vi "Modify_Image_Histogram-1.vi"(4 "[IN] Parameter":sgl format="%.2f", 6 "[IN] Operator":T4(ring), 7 "# channel":u8, 8 "error IN":errorcluster, 9 "[IN] Filtering Settings":T2, 11 "[IN] LoG Processed Image":T3) -> (0 "error OUT":errorcluster, 1 "[OUT] Filtering Settings":T2, 2 "[OUT] Histogram":T1 {"Incremental Value" format="%.2f"; "Starting Value" format="%.2f"}, 3 "[OUT] Histogram Modified Image":T3)   [LabVIEW 2013]
doc: "This subVI modifies image through various mathlookup operations (see the built-in function \"IMAQ MathLookup\")"
uses:
  <vilib>/vision/Image Controls.llb/IMAQ Image.ctl
  <vilib>/vision/NI_Vision_Development_Module.lvlib
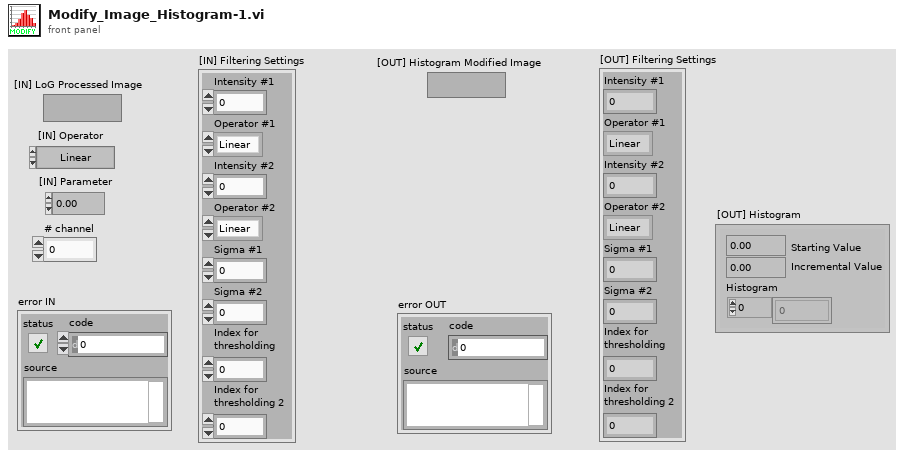
[diagram p1: front panel]
types:
  T1 = cluster{"Starting Value":sgl, "Incremental Value":sgl, "Histogram":u32[]}
  T2 = cluster{"Intensity #1":sgl, "Operator #1":enum32{"Linear", "Log", "Exp", "Square", "Square root", "Power X", "Power 1/X"}, "Intensity #2":sgl, "Operator #2":enum32{"Linear", "Log", "Exp", "Square", "Square root", "Power X", "Power 1/X"}, "Sigma #1":dbl, "Sigma #2":dbl, "Index for \nthresholding":u8, "Index for \nthresholding 2":u8}
  T3 = typedef "IMAQ Image.ctl" = refnum<image>
  T4 = enum32{"Linear", "Log", "Exp", "Square", "Square root", "Power X", "Power 1/X"}
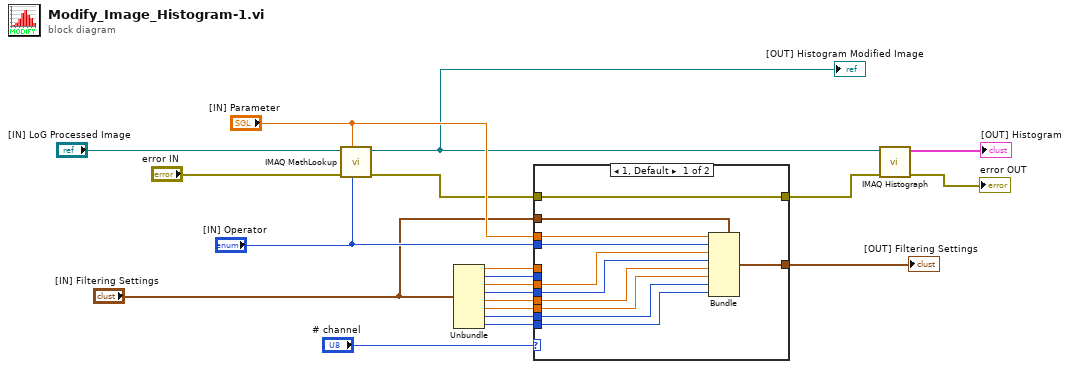
[diagram p0: block diagram]
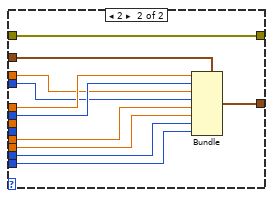
[diagram p2: hidden frame]
diagram:
  n1 = call "IMAQ MathLookup"("Operator"="[IN] Operator", "X Value"="[IN] Parameter", "error in (no error)"="error IN", "Image Src"="[IN] LoG Processed Image") -> ("error out"=w4:errorcluster, "Image Dst Out"=w5:T3)  [unwired: 6 in]
  "[OUT] Histogram Modified Image" <- w5
  n2 = Unbundle("[IN] Filtering Settings") -> ("Intensity #1"=w17:sgl, "Operator #1"=w16:T4, "Intensity #2"=w15:sgl, "Operator #2"=w14:T4, "Sigma #1"=w10:dbl, "Sigma #2"=w9:dbl, "Index for \nthresholding"=w8:u8, "Index for \nthresholding 2"=w7:u8)
  n3 = case shown="1, Default" "# channel" {
    tunnel: w17 -> [_ w41]
    tunnel: w16 -> [_ w40]
    tunnel: w15 -> [w27 _]
    tunnel: w14 -> [w26 _]
    tunnel: "[IN] Parameter" -> [w30 w39]
    tunnel: "[IN] Operator" -> [w28 w38]
    tunnel: "[IN] Filtering Settings" -> [w31 w42]
    tunnel: w10 -> [w25 w35]
    tunnel: w9 -> [w24 w34]
    tunnel: w8 -> [w23 w36]
    tunnel: w7 -> [w22 w37]
    tunnel: [w29 w33] -> w6
    tunnel: w4 -> [w21 w32]
    tunnel: [w21 w32] -> w3
    frame 1, Default {
      n4 = Bundle(cluster=w31, "Intensity #1"=w30, "Operator #1"=w28, "Intensity #2"=w27, "Operator #2"=w26, "Sigma #1"=w25, "Sigma #2"=w24, "Index for \nthresholding"=w23, "Index for \nthresholding 2"=w22) -> (w29:T2)
    }
    frame 2 {
      n5 = Bundle(cluster=w42, "Intensity #1"=w41, "Operator #1"=w40, "Intensity #2"=w39, "Operator #2"=w38, "Sigma #1"=w35, "Sigma #2"=w34, "Index for \nthresholding"=w36, "Index for \nthresholding 2"=w37) -> (w33:T2)
    }
  }
  "[OUT] Filtering Settings" <- w6
  n6 = call "IMAQ Histograph"("error in (no error)"=w3, "Image"=w5) -> ("error out"=→"error OUT":errorcluster, "Histogram Graph"=→"[OUT] Histogram":T1)  [unwired: 6 in, 2 out]
